vi "Needle_controller_tester_stream.vi"() -> ()   [LabVIEW 2018]
uses:
  <vilib>/Analysis/baseanly.llb/Mean (DBL).vi
  <vilib>/Analysis/baseanly.llb/A x Vector.vi
  <vilib>/Analysis/NI_AALBase.lvlib
  <vilib>/ptbypt/NI_PtbyPt.lvlib
panel:
  out "Time":i32=3286291
  out "Encoder Data":cluster{"X":sgl, "Y":sgl, "X":sgl}
  out "Execution ms":dbl=10.248249999995096 format="%0.2f"
  out "Sample rate (Hz)":dbl=97.57763520605747 format="%0.2f"
  out "FT Data":T1={"X (N)"=-0.0031637721176096534, "Y (N)"=0.0020654385557108412, "Z (N)"=-0.0012890235481179957, "X (Nm)"=0.011304788564686419, "Y (Nm)"=0.006585666954038061, "Z (Nm)"=0.015090134978294145}
  in  "Stop Stream":bool
  out "Waveform Chart":T2(graph)={"[0]"=-0.0031637721176096534, "[1]"=0.0020654385557108412, "[2]"=-0.0012890235481179957, "[3]"=0.011304788564686419, "[4]"=0.006585666954038061, "[5]"=0.015090134978294145, "[6]"=0.0, "[7]"=0.0, "[8]"=0.0}
  in  "Start Stream":bool
  out "Error Code":T3(ring)
  out "Return FID":u8=2
  out "FID":u8=6
  in  "IP Address":string="192.168.5.101"
  out "error out":errorcluster
  in  "Stop":bool
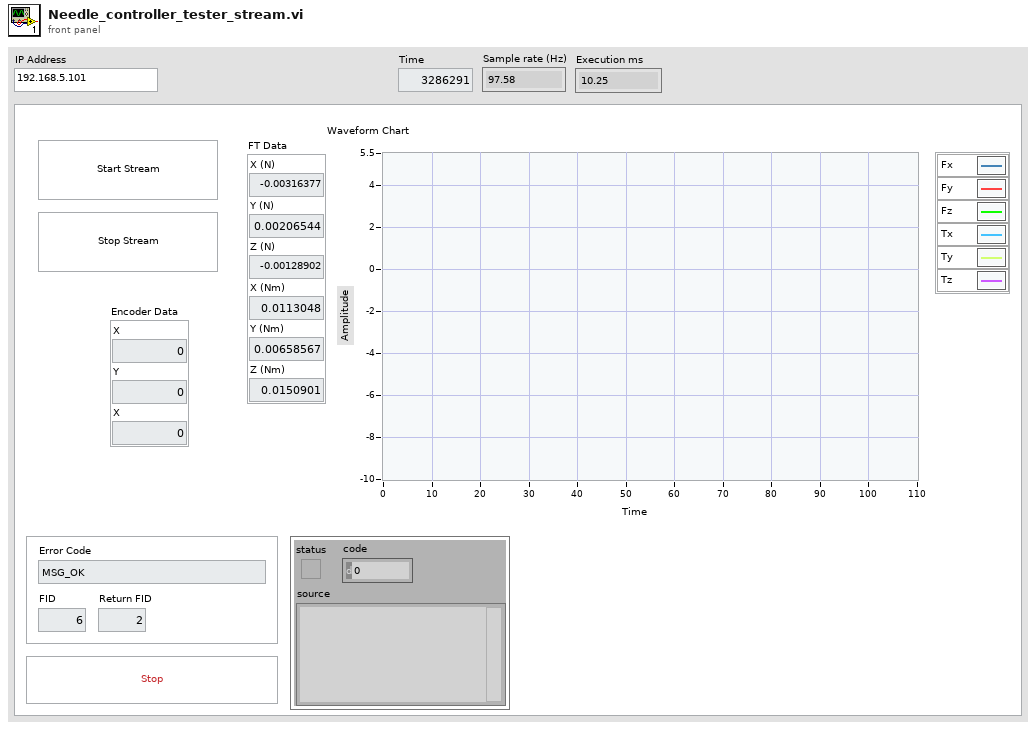
[diagram p1: front panel]
types:
  T1 = cluster{"X (N)":dbl, "Y (N)":dbl, "Z (N)":dbl, "X (Nm)":dbl, "Y (Nm)":dbl, "Z (Nm)":dbl}
  T2 = cluster{"[0]":dbl, "[1]":dbl, "[2]":dbl, "[3]":dbl, "[4]":dbl, "[5]":dbl, "[6]":dbl, "[7]":dbl, "[8]":dbl}
  T3 = enum8{"MSG_OK", "MSG_ERROR_NOT_SUPPORTED", "MSG_ERROR_SENSOR_DISCONNECTED", "MSG_ERROR_READING_PENDING"}
  T4 = cluster{"[0]":dbl, "[1]":dbl, "[2]":dbl, "[3]":dbl, "[4]":dbl, "[5]":dbl, "[6]":dbl, "[7]":dbl, "[8]":dbl}[]
  T5 = enum16{"Default", "Start Acquisition Stream", "Stop Acquisition Stream", "Read"}
  T6 = enum16{"big-endian, network order", "native, host order", "little-endian"}
  T7 = cluster{i32, cluster{sgl, sgl, sgl, sgl, sgl, sgl}, cluster{sgl, sgl, sgl}}
  T8 = cluster{"pumpState":i32, "suppliedVolume_ml":sgl, "flowRate_mlmin":sgl, "home":i32, "port":i32}
  T9 = cluster{"connection ID":refnum<k5>, "header length":u16}
  T10 = cluster{"header":cluster{"length":u16, "fid":u8, "error":u8}}
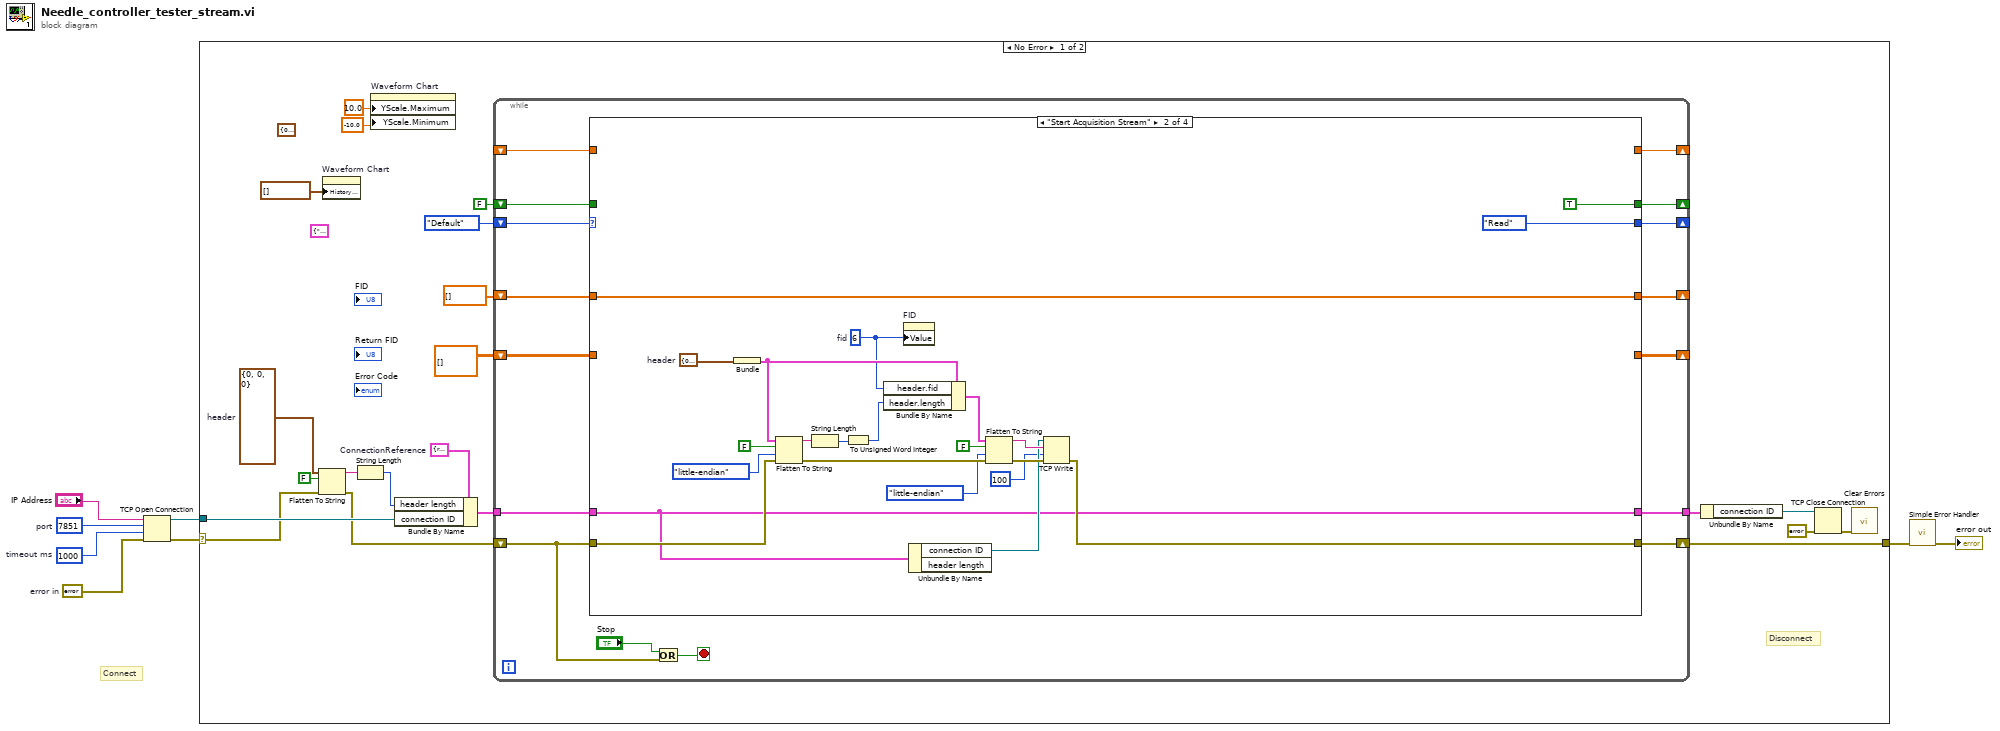
[diagram p0: block diagram]
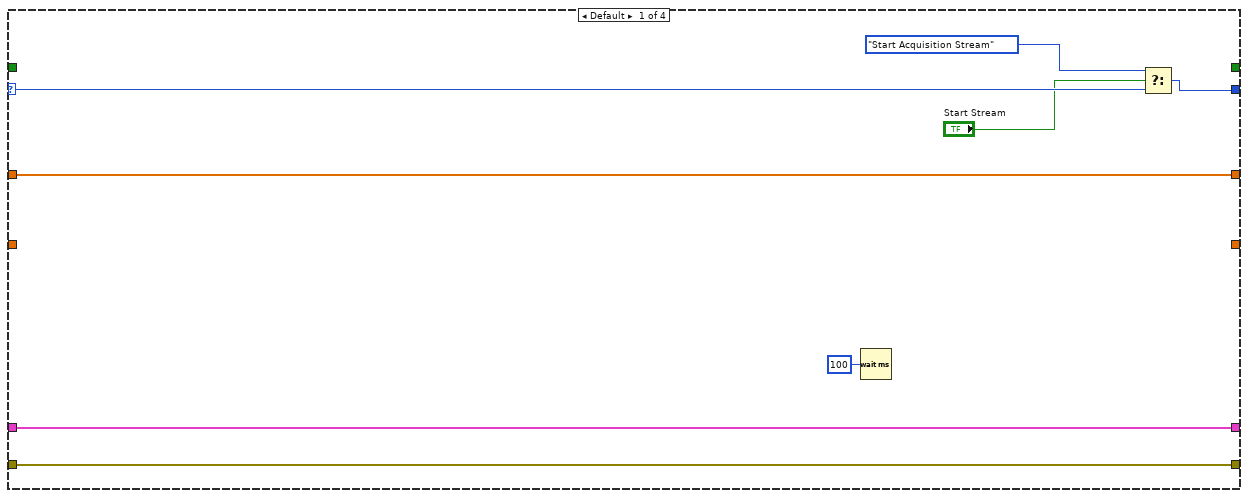
[diagram p2: hidden frame]
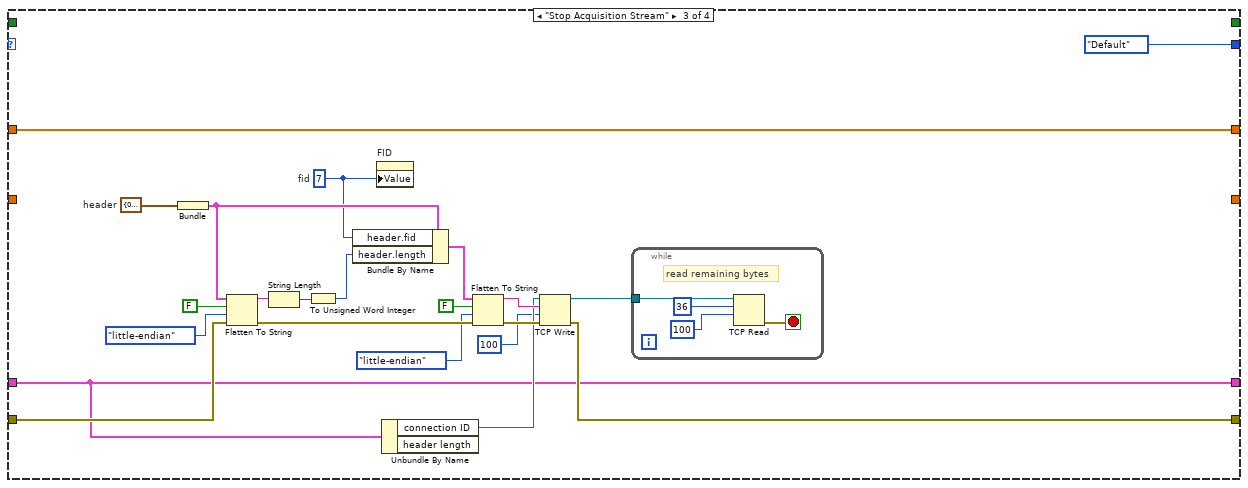
[diagram p3: hidden frame]
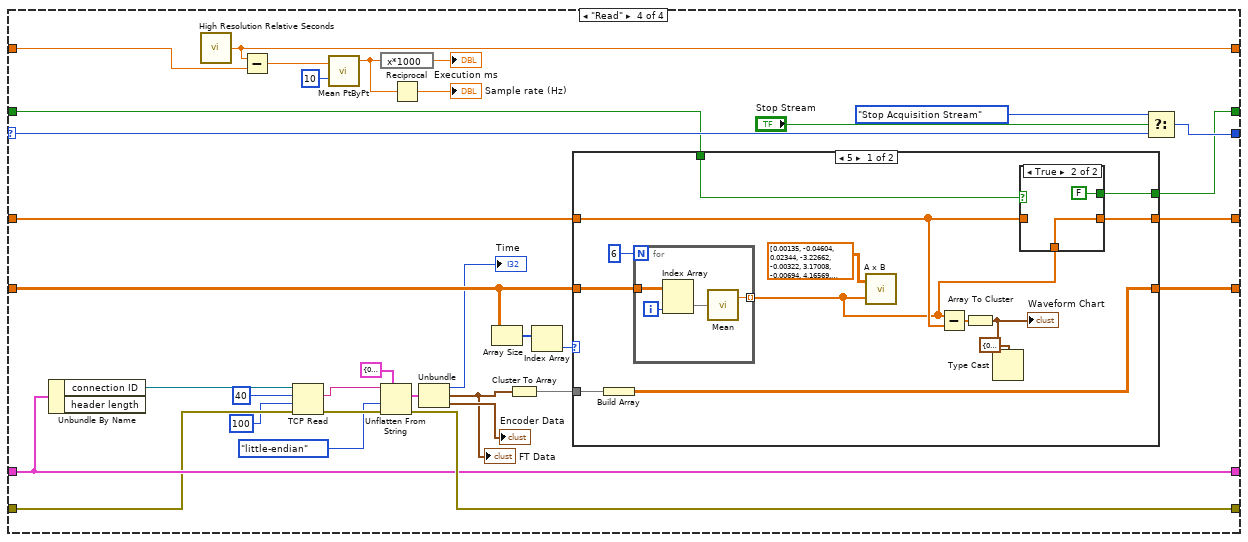
[diagram p4: hidden frame]
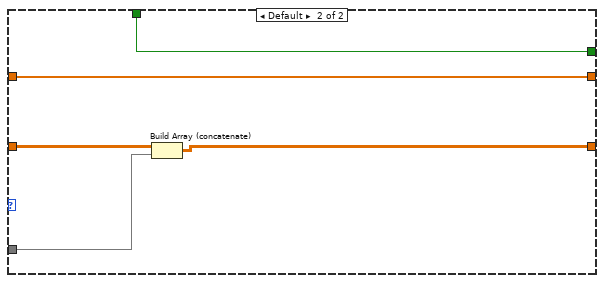
[diagram p6: hidden frame]
diagram:
  w6 = errorcluster {"status"=FALSE, "code"=0, "source"=""}  # error in
  w7 = 1000  # timeout ms
  w8 = u16 7851  # port
  # "Connect"
  n1 = TCP Open Connection(address="IP Address", remote port or service name=w8, timeout ms (60000)=w7, error in (no error)=w6) -> (connection ID=w5:refnum<k5>, error out=w1:errorcluster)  [unwired: 1 in]
  n2 = case shown="No Error" w1 {
    selector: w1 -> [w18 w161]
    tunnel: w5 -> [w25 _]
    tunnel: [w16 w161] -> w2
    frame No Error {
      (unwired) cluster{"axis":string, "stepPeriod (ms)":string} {"axis"="", "stepPeriod (ms)"=""} ("Return Motor Config")
      (unwired) T8 {"pumpState"=0, "suppliedVolume_ml"=0.0, "flowRate_mlmin"=0.0, "home"=0, "port"=0} ("Status")
      w24 = cluster{"length":u16, "fid":u8, "error":u8} {"length"=0, "fid"=0, "error"=0}  # header
      w26 = T9 {"connection ID"=refnum, "header length"=0}  # ConnectionReference
      # "Disconnect"
      n3 = Flatten To String(anything=w24, prepend array or string size? (T)=FALSE, error in (no error)=w18) -> (data string=w22:string, error out=w19:errorcluster)  [unwired: 1 in, 1 out]
      n4 = property on="Waveform Chart" class="WFChart (strict)"("History Data"=T4 []) -> ()  [unwired: 2 in, 2 out]
      n5 = String Length(string=w22) -> (length=w21:i32)
      n6 = property on="Waveform Chart" class="WFChart (strict)"("YScale.Maximum"=10.0 ("Y Scale.Range:Maximum"), "YScale.Minimum"=-10.0 ("Y Scale.Range:Minimum")) -> ()  [unwired: 2 in, 2 out]
      n7 = Bundle By Name(cluster=w26, "header length"=w21, "connection ID"=w25) -> (w20:T9)
      n8 = while {
        tunnel: w20 -> [w40]
        shift-right: [w42] -> w16
        shift-left: w19 -> [w43]
        tunnel: [w41] -> w17
        shift-right: [w39] -> _
        shift-left: T5."Default" ("Case") -> [w38]
        shift-right: [w37] -> _
        shift-left: sgl[][] [] ("appended array") -> [w36]
        shift-right: [w35] -> _
        shift-left: dbl[] [] ("A x Vector") -> [w34]
        shift-right: [w33] -> _
        shift-left: FALSE -> [w32]
        shift-right: [w31] -> _
        shift-left: _ -> [w30]
        stop <- w45 stop-if-true
        n9 = case shown="\"Start Acquisition Stream\"" w38 {
          selector: w38 -> [w53 _ _ w126]
          tunnel: w43 -> [w47 w60 w82 w127]
          tunnel: [w47 w59 w81 w132] -> w42
          tunnel: [w48 w58 w80 w131] -> w41
          tunnel: w40 -> [w48 w58 w80 w131]
          tunnel: [w51 T5."Read" ("Case") T5."Default" ("t") w128] -> w39
          tunnel: [_ _ _ w125] -> w37
          tunnel: w36 -> [_ _ _ w123]
          tunnel: [w46 w55 w77 w117] -> w35
          tunnel: w34 -> [w46 w55 w77 w116]
          tunnel: [_ TRUE _ w114] -> w33
          tunnel: w32 -> [_ _ _ w115]
          tunnel: [_ _ _ w112] -> w31
          tunnel: w30 -> [_ _ _ w113]
          frame Default {
            n10 = Wait (ms)(milliseconds to wait=u32 100) -> ()  [unwired: 1 out]
            n11 = Select(t=T5."Start Acquisition Stream", s="Start Stream", f=w53) -> (s? t:f=w51:T5)
          }
          frame "Start Acquisition Stream" {
            w65 = cluster{"length":u16, "fid":u8, "error":u8} {"length"=0, "fid"=0, "error"=0}  # header
            w57 = u8 6  # fid
            n12 = Bundle("header"=w65) -> (w71:T10)  [unwired: 1 in]
            n13 = Flatten To String(anything=w71, prepend array or string size? (T)=FALSE, byte order (0:big-endian, network order)=T6."little-endian", error in (no error)=w60) -> (data string=w69:string, error out=w70:errorcluster)  [unwired: 1 out]
            n14 = String Length(string=w69) -> (length=w68:i32)
            n15 = To Unsigned Word Integer(number=w68) -> (unsigned 16bit integer=w67:u16)
            n16 = Bundle By Name(cluster=w71, "header.fid"=w57, "header.length"=w67) -> (w72:T10)
            n17 = property on="FID" class="DigNum (strict)"("Value"=w57) -> ()  [unwired: 2 in, 2 out]
            n18 = Unbundle By Name(w58) -> ("connection ID"=w63:refnum<k5>)  [unwired: 1 out]
            n19 = Flatten To String(anything=w72, prepend array or string size? (T)=FALSE, byte order (0:big-endian, network order)=T6."little-endian", error in (no error)=w70) -> (data string=w74:string, error out=w75:errorcluster)  [unwired: 1 out]
            n20 = TCP Write(connection ID=w63, data in=w74, error in (no error)=w75, 9:100 ("timeout ms (25000)")) -> (error out=w59:errorcluster)  [unwired: 2 out]
          }
          frame "Stop Acquisition Stream" {
            w87 = cluster{"length":u16, "fid":u8, "error":u8} {"length"=0, "fid"=0, "error"=0}  # header
            w79 = u8 7  # fid
            n21 = Bundle("header"=w87) -> (w93:T10)  [unwired: 1 in]
            n22 = Flatten To String(anything=w93, prepend array or string size? (T)=FALSE, byte order (0:big-endian, network order)=T6."little-endian", error in (no error)=w82) -> (data string=w91:string, error out=w92:errorcluster)  [unwired: 1 out]
            n23 = String Length(string=w91) -> (length=w90:i32)
            n24 = To Unsigned Word Integer(number=w90) -> (unsigned 16bit integer=w89:u16)
            n25 = Bundle By Name(cluster=w93, "header.fid"=w79, "header.length"=w89) -> (w94:T10)
            n26 = property on="FID" class="DigNum (strict)"("Value"=w79) -> ()  [unwired: 2 in, 2 out]
            n27 = Unbundle By Name(w80) -> ("connection ID"=w85:refnum<k5>)  [unwired: 1 out]
            n28 = Flatten To String(anything=w94, prepend array or string size? (T)=FALSE, byte order (0:big-endian, network order)=T6."little-endian", error in (no error)=w92) -> (data string=w96:string, error out=w97:errorcluster)  [unwired: 1 out]
            n29 = TCP Write(connection ID=w85, data in=w96, error in (no error)=w97, 9:100 ("timeout ms (25000)")) -> (connection ID out=w76:refnum<k5>, error out=w81:errorcluster)  [unwired: 1 out]
            n30 = while {
              tunnel: w76 -> [w99]
              stop <- w98 stop-if-true
              # "read remaining bytes"
              n31 = TCP Read(connection ID=w99, bytes to read=36, 9:100 ("timeout ms (25000)")) -> (error out=w98:errorcluster)  [unwired: 2 in, 2 out]
            }
          }
          frame "Read" {
            n32 = Unbundle By Name(w131) -> ("connection ID"=w135:refnum<k5>)  [unwired: 1 out]
            n33 = call <vilib>:"High Resolution Relative Seconds.vi"() -> ("relative seconds"=w112:dbl)
            n34 = Subtract(x=w112, y=w113) -> (x-y=w110:dbl)
            n35 = TCP Read(connection ID=w135, bytes to read=40, error in (no error)=w127, 9:100 ("timeout ms (25000)")) -> (data out=w120:string, error out=w134:errorcluster)  [unwired: 1 in, 1 out]
            n36 = call <vilib>:"Mean PtByPt.vi"("x"=w110, "sample length"=10) -> ("mean"=w108:dbl)  [unwired: 2 in, 1 out]
            n37 = expression code="x*1000"(w108) -> (→"Execution ms":dbl)
            n38 = Unflatten From String(type=T7 {0, {0.0, 0.0, 0.0, 0.0, 0.0, 0.0}, {0.0, 0.0, 0.0}}, binary string=w120, byte order (0:big-endian, network order)=T6."little-endian", error in (no error)=w134) -> (value=w105:T7, error out=w132:errorcluster)  [unwired: 1 in, 1 out]
            n39 = Reciprocal(x=w108) -> (1/x=→"Sample rate (Hz)":dbl)
            n40 = Unbundle(w105) -> (→"Time":i32, w102:cluster{sgl, sgl, sgl, sgl, sgl, sgl}, →"Encoder Data":cluster{sgl, sgl, sgl})
            "FT Data" <- w102
            n41 = Array Size(array=w123) -> (size(s)=w122:i32[])
            n42 = Cluster To Array(cluster=w102) -> (array=w124:sgl[])
            n43 = Index Array(array=w122) -> (element=w121:i32)  [unwired: 1 in]
            n44 = case shown="5" w121 {
              tunnel: w123 -> [w143 w158]
              tunnel: [w144 w159] -> w125
              tunnel: w124 -> [w137 w160]
              tunnel: [w148 w157] -> w117
              tunnel: w116 -> [w147 w157]
              tunnel: w115 -> [w146 w156]
              tunnel: [w145 w156] -> w114
              frame 5 {
                n45 = Build Array(w137) -> (w144:sgl[][])
                n46 = for {
                  N: 6 -> [_]
                  tunnel: w143 -> [w151]
                  tunnel: [w152] -> w136 mode=indexing
                  i -> [w150]
                  n47 = Index Array(array=w151, index (col)=w150) -> (element=w149:sgl[])  [unwired: 1 in]
                  n48 = call-poly <vilib>:"Mean.vi"("X"=w149) -> ("mean"=w152:dbl)  [unwired: 1 out]
                }
                n49 = call-poly <vilib>:"A x B.vi"("Vector"=w136, "A"=dbl[][] [[0.00135, -0.04604, 0.02344, -3.22662, -0.00322, 3.17008], [-0.00694, 4.16569, 0.02971, -1.87643, 0.02738, -1.79608], [3.69182, 0.02713, 3.83425, -0.03329, 3.65801, -0.067], [0.15408, 25.37956, 21.34115, -11.71178, -20.50426, -10.51265], [-23.9405, 0.07684, 12.2178, 19.58172, 12.22442, -19.60731], [0.09832, 17.49271, -0.32435, 15.76607, -0.09154, 15.24495]] ("Calibration Matrix")) -> ()  [unwired: 2 out]
                n50 = Subtract(x=w136, y=w147) -> (x-y=w142:dbl[])
                n51 = Array To Cluster(array=w142) -> (cluster=w140:T2)
                "Waveform Chart" <- w140
                n52 = Type Cast(type=T1 {"X (N)"=0.0, "Y (N)"=0.0, "Z (N)"=0.0, "X (Nm)"=0.0, "Y (Nm)"=0.0, "Z (Nm)"=0.0} ("Data"), x=w140) -> ()  [unwired: 1 out]
                n53 = case shown="True" w146 {
                  tunnel: [w153 w155] -> w148
                  tunnel: w136 -> [_ w155]
                  tunnel: w147 -> [w153 _]
                  tunnel: [_ FALSE] -> w145
                  frame False {
                  }
                  frame True {
                  }
                }
              }
              frame Default {
                n54 = Build Array (concatenate)(w158, w160) -> (w159:sgl[][])
              }
            }
            n55 = Select(t=T5."Stop Acquisition Stream", s="Stop Stream", f=w126) -> (s? t:f=w128:T5)
          }
        }
        n56 = Or(x="Stop", y=w43) -> (x .or. y?=w45:bool)
      }
      n57 = Unbundle By Name(w17) -> ("connection ID"=w27:refnum<k5>)
      n58 = TCP Close Connection(connection ID=w27, error in (no error)=errorcluster {"status"=FALSE, "code"=0, "source"=""}) -> (error out=w28:errorcluster)  [unwired: 1 in, 1 out]
      n59 = call <vilib>:"Clear Errors.vi"("error in (no error)"=w28) -> ()  [unwired: 5 in, 2 out]
    }
    frame Error {
    }
  }
  n60 = call <vilib>:"Simple Error Handler.vi"("error in (no error)"=w2) -> ("error out"=→"error out":errorcluster)  [unwired: 4 in, 4 out]
